vi "Generate Project + Actor Name.vi"(11 "Actor in":refnum<class "Actor.lvclass">) -> (3 "concatenated string":string)   [LabVIEW 2015, in "Actor.lvclass"]
uses:
  Actor.lvclass
  Actor.lvclass/Actor.ctl
  Application Info/App Info.lvlib
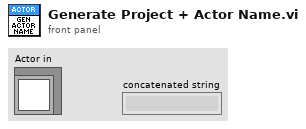
[diagram p1: front panel]
types:
  T1 = typedef "App Info.lvlib/Core Data.ctl" = cluster{"Version":string, "Misc Info":string, "Name":string, "Name 2":string}
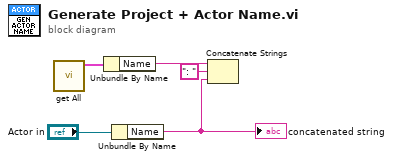
[diagram p0: block diagram]
diagram:
  n1 = call "get All.vi"() -> ("Data out"=w3:T1)  [unwired: 10 in, 1 out]
  n2 = Unbundle By Name(w3) -> ("Name"=w4:string)
  n3 = Unbundle By Name("Actor in") -> ("Name"=w1:string)
  "concatenated string" <- w1
  n4 = Concatenate Strings(w4, ": " ("string"), w1) -> ()  [unwired: 1 out]
